vi "Modify Item Owner.vi"(8 "error in (no error)":errorcluster, 9 "New Parent Fully Qualified Name":string, 10 "UniqueName Object":refnum<class "UniqueName.lvclass">, 11 "Registry in":refnum<data-value>) -> (0 "error out":errorcluster, 1 "Modified":bool, 2 "UniqueName Object out":refnum<class "UniqueName.lvclass">, 3 "Registry":refnum<data-value>)   [LabVIEW 2014, in "UniqueName.lvlib" / "NameRegistry.lvclass"]
uses:
  NameRegistry.lvclass
  UniqueNameClass/UniqueName.lvclass
  UniqueNameClass/UniqueName.lvclass/UniqueName.ctl
  NameRegistry.lvclass/NameRegistry.ctl
  UniquenessCriteria/UniquenessCriteria.lvclass/UniquenessCriteria.ctl
  UniqueNameClass/Key.ctl
  Delimiter/DelimiterToStringRepresentation.vi
  <vilib>/Utility/error.llb/Trim Whitespace.vi
  UniquenessCriteria/UniquenessCriteria.lvclass
  StringIncrement/StringIncrement.lvclass
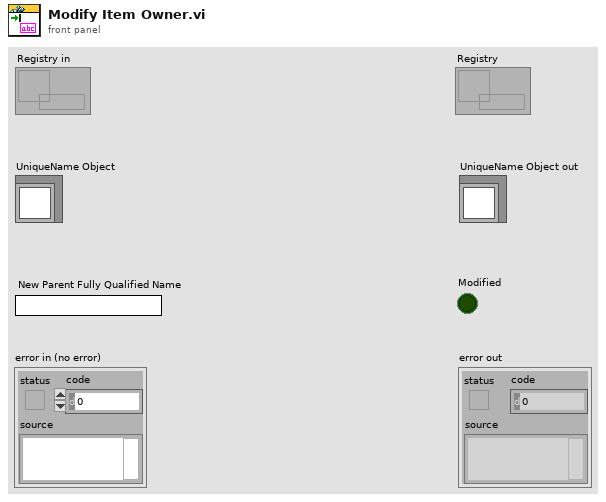
[diagram p1: front panel]
types:
  T1 = typedef "UniqueName.lvlib/UniqueName.lvclass/Key.ctl" = enum16{"Fully Qualified Name", "Unique Name", "Given Name", "Parent Fully Qualified Name"}
  T2 = typedef "UniqueName.lvlib/UniquenessCriteria.lvclass/Criteria.ctl" = enum16{"Globally-Unique Fully Qualified Name", "Globally-Unique Name"}
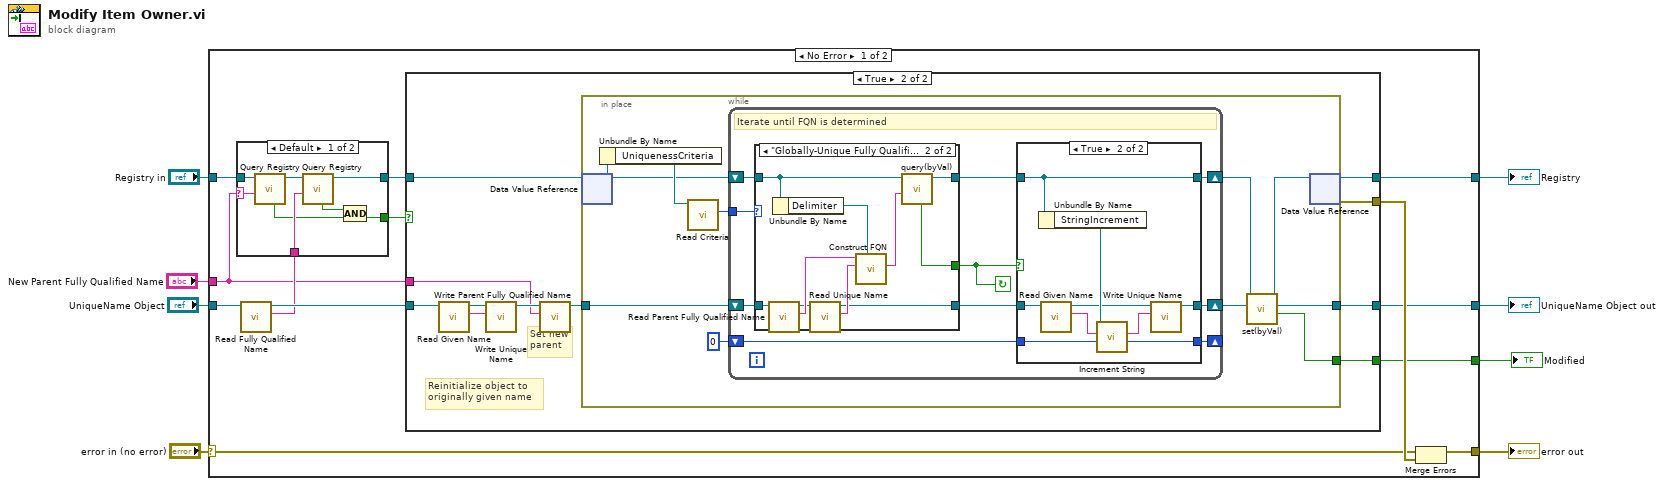
[diagram p0: block diagram]
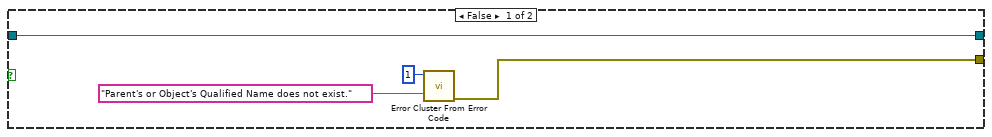
[diagram p2: hidden frame]
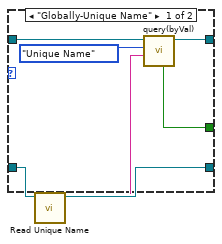
[diagram p4: hidden frame]
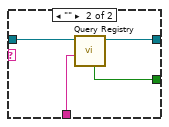
[diagram p5: hidden frame]
diagram:
  n1 = case shown="No Error" "error in (no error)" {
    selector: "error in (no error)" -> [w19 w99]
    tunnel: "Registry in" -> [w17 w100]
    tunnel: [w21 w100] -> w7
    tunnel: [w18 w99] -> w5
    tunnel: "New Parent Fully Qualified Name" -> [w10 _]
    tunnel: [w14 w98] -> w3
    tunnel: "UniqueName Object" -> [w13 w98]
    tunnel: [w9 _] -> w1
    frame No Error {
      n2 = call "Read Fully Qualified Name.vi"("UniqueName in"=w13) -> ("Fully Qualified Name"=w11:string, "UniqueName out"=w12:refnum<class "UniqueName.lvclass">)  [unwired: 9 in]
      n3 = case shown="Default" w10 {
        selector: w10 -> [w92 _]
        tunnel: w17 -> [w93 w95]
        tunnel: [w90 w97] -> w16
        tunnel: [w87 w94] -> w15
        tunnel: w11 -> [w89 w96]
        frame Default {
          n4 = call "Query Registry.vi"("Search string"=w92, "Registry in"=w93) -> ("Registry"=w91:refnum<data-value>, "found?"=w88:bool)  [unwired: 5 in, 3 out]
          n5 = call "Query Registry.vi"("Search string"=w89, "Registry in"=w91) -> ("Registry"=w90:refnum<data-value>, "found?"=w86:bool)  [unwired: 5 in, 3 out]
          n6 = Compound Arithmetic op=AND(w86, w88) -> (w87:bool)
        }
        frame "" {
          n7 = call "Query Registry.vi"("Search string"=w96, "Registry in"=w95) -> ("Registry"=w97:refnum<data-value>, "found?"=w94:bool)  [unwired: 5 in, 3 out]
        }
      }
      n8 = case shown="True" w15 {
        tunnel: [w25 w36] -> w21
        tunnel: [w23 w35] -> w20
        tunnel: w16 -> [w25 w32]
        tunnel: w10 -> [_ w33]
        tunnel: [_ w30] -> w14
        tunnel: w12 -> [_ w29]
        tunnel: [_ w26] -> w9
        frame False {
          n9 = call <vilib>:"Error Cluster From Error Code.vi"("error message (\"\")"="Parent's or Object's Qualified Name does not exist." ("error message (\"\")"), "error code (0)"=1) -> ("error out"=w23:errorcluster)  [unwired: 7 in]
        }
        frame True {
          # "Set new\nparent"
          # "Reinitialize object to\noriginally given name"
          n10 = call "Read Given Name.vi"("UniqueName in"=w29) -> ("Given Name"=w28:string, "UniqueName out"=w27:refnum<class "UniqueName.lvclass">)  [unwired: 9 in]
          n11 = call "Write Unique Name.vi"("Unique Name"=w28, "UniqueName in"=w27) -> ("UniqueName out"=w34:refnum<class "UniqueName.lvclass">)  [unwired: 9 in]
          n12 = call "Write Parent Fully Qualified Name.vi"("Parent Fully Qualified Name"=w33, "UniqueName in"=w34) -> ("UniqueName out"=w31:refnum<class "UniqueName.lvclass">)  [unwired: 9 in]
          n13 = in-place {
            in-place-border: w31 -> [w44]
            in-place-border: [w41] -> w30
            in-place-border: [w38] -> w26
            n14 = in-place-dvr #1(w32) -> (w43:refnum<class "NameRegistry.lvclass">)  [unwired: 1 out]
            n15 = Unbundle By Name(w43) -> ("UniquenessCriteria"=w46:refnum<class "UniquenessCriteria.lvclass">)
            n16 = call "Read Criteria.vi"("UniquenessCriteria in"=w46) -> ("Criteria"=w45:T2)  [unwired: 9 in, 1 out]
            n17 = while {
              tunnel: w45 -> [w56]
              shift-right: [w54] -> w42
              shift-left: w44 -> [w53]
              shift-right: [w49] -> w40
              shift-left: w43 -> [w51]
              shift-right: [w48] -> _
              shift-left: u32 0 ("Incremented Numeric") -> [w47]
              stop <- w52 continue-if-true
              # "Iterate until FQN is determined"
              n18 = case shown="\"Globally-Unique Fully Qualified Name\"" w56 {
                tunnel: [w72 w79] -> w52
                tunnel: w53 -> [w75 w83]
                tunnel: [w74 w81] -> w55
                tunnel: w51 -> [w73 w77]
                tunnel: [w69 w78] -> w50
                frame "Globally-Unique Name" {
                  n19 = call "Read Unique Name.vi"("UniqueName in"=w75) -> ("Unique Name"=w70:string, "UniqueName out"=w74:refnum<class "UniqueName.lvclass">)  [unwired: 9 in]
                  n20 = call "query(byVal).vi"("Search string"=w70, "Search Key (FQN)"=Key."Unique Name" ("Key (FQN)"), "Instance"=w73) -> ("Instance"=w69:refnum<class "NameRegistry.lvclass">, "found?"=w72:bool)  [unwired: 5 in, 2 out]
                }
                frame "Globally-Unique Fully Qualified Name" {
                  n21 = call "Read Parent Fully Qualified Name.vi"("UniqueName in"=w83) -> ("Parent Fully Qualified Name"=w85:string, "UniqueName out"=w82:refnum<class "UniqueName.lvclass">)  [unwired: 9 in]
                  n22 = Unbundle By Name(w77) -> ("Delimiter"=w76:refnum<class "Delimiter.lvclass">)
                  n23 = call "Read Unique Name.vi"("UniqueName in"=w82) -> ("Unique Name"=w84:string, "UniqueName out"=w81:refnum<class "UniqueName.lvclass">)  [unwired: 9 in]
                  n24 = call "Construct FQN.vi"("Delimiter"=w76, "Name"=w84, "Parent FQN"=w85) -> ("FQN"=w80:string)  [unwired: 8 in]
                  n25 = call "query(byVal).vi"("Search string"=w80, "Instance"=w77) -> ("Instance"=w78:refnum<class "NameRegistry.lvclass">, "found?"=w79:bool)  [unwired: 6 in, 2 out]
                }
              }
              n26 = case shown="True" w52 {
                tunnel: w55 -> [w59 w64]
                tunnel: [w59 w68] -> w54
                tunnel: w50 -> [w58 w66]
                tunnel: [w58 w66] -> w49
                tunnel: [w57 w61] -> w48
                tunnel: w47 -> [w57 w60]
                frame False {
                  # "Name already unique"
                }
                frame True {
                  n27 = Unbundle By Name(w66) -> ("StringIncrement"=w65:refnum<class "StringIncrement.lvclass">)
                  n28 = call "Read Given Name.vi"("UniqueName in"=w64) -> ("Given Name"=w63:string, "UniqueName out"=w62:refnum<class "UniqueName.lvclass">)  [unwired: 9 in]
                  n29 = call "Increment String.vi"("Numeric"=w60, "Input String"=w63, "StringIncrement"=w65) -> ("Incremented Numeric"=w61:u32, "Incremented String"=w67:string)  [unwired: 7 in]
                  n30 = call "Write Unique Name.vi"("Unique Name"=w67, "UniqueName in"=w62) -> ("UniqueName out"=w68:refnum<class "UniqueName.lvclass">)  [unwired: 9 in]
                }
              }
            }
            n31 = call "set(byVal).vi"("UniqueName in"=w42, "NameRegistry in"=w40) -> ("Replaced?"=w38:bool, "UniqueName out"=w41:refnum<class "UniqueName.lvclass">, "NameRegistry out"=w39:refnum<class "NameRegistry.lvclass">)  [unwired: 7 in]
            n32 = in-place-dvr #1(w39) -> (w36:refnum<data-value>, w35:errorcluster)
          }
        }
      }
      n33 = Merge Errors(w19, w20) -> (w18:errorcluster)
    }
    frame Error {
    }
  }
  "error out" <- w5
  "Registry" <- w7
  "UniqueName Object out" <- w3
  "Modified" <- w1
